vi "WriteBatches.vi"(8 "Variable Parameter Value":dbl, 9 "Image Number":dbl, 10 "Scan Name":string, 11 "Raw Data Folder":path) -> ()   [LabVIEW 2013]
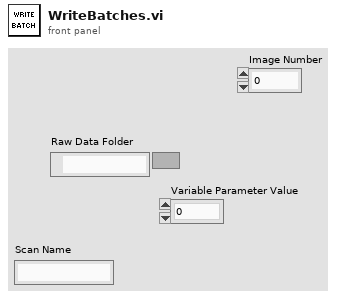
[diagram p1: front panel]
types:
  T1 = enum16{"open", "replace", "create", "open or create", "replace or create", "replace or create with confirmation"}
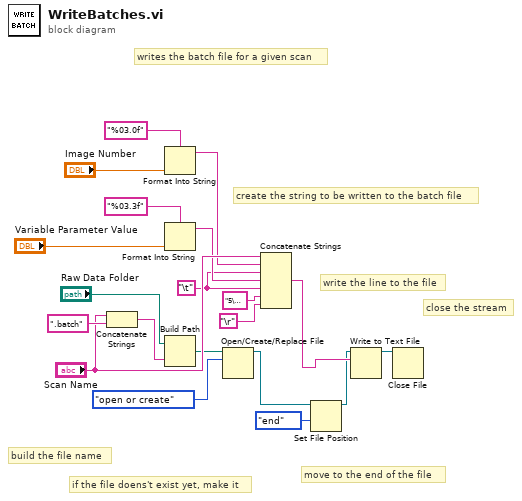
[diagram p0: block diagram]
diagram:
  w11 = "\t"
  # "close the stream"
  # "write the line to the file"
  # "create the string to be written to the batch file"
  # "move to the end of the file"
  # "if the file doens't exist yet, make it"
  # "build the file name"
  # "writes the batch file for a given scan"
  n1 = Concatenate Strings("Scan Name", ".batch" ("string")) -> (w19:string)
  n2 = Format Into String(format string="%03.0f", "Image Number") -> (resulting string=w15:string)  [unwired: 2 in, 1 out]
  n3 = Format Into String(format string="%03.3f", "Variable Parameter Value") -> (resulting string=w12:string)  [unwired: 2 in, 1 out]
  n4 = Build Path(base path="Raw Data Folder", name or relative path=w19) -> (appended path=w7:path)
  n5 = Open/Create/Replace File(file path (use dialog)=w7, operation (0:open)=T1."open or create") -> (refnum out=w2:refnum<file>)  [unwired: 4 in, 2 out]
  n6 = Concatenate Strings("Scan Name", w15, w11, w12, w11, "5\t2chscopeoff\t2.53767\t-1.76423\t10\t25\t0\t0\t0.021406\twavemeteroff" ("string"), "\r") -> (w4:string)
  n7 = Set File Position(refnum=w2, from (0:start)=enum16{"start", "end", "current"}."end") -> (refnum out=w3:refnum<file>)  [unwired: 2 in, 1 out]
  n8 = Write to Text File(file (use dialog)=w3, text=w4) -> (refnum out=w5:refnum<file>)  [unwired: 2 in, 2 out]
  n9 = Close File(refnum=w5) -> ()  [unwired: 1 in, 2 out]
